vi "JoystickReader.vi"(8 "Reset":bool, 11 "Refnum in":refnum<k20>) -> (0 "L4 [deg]":sgl, 1 "L3 [0~100]":sgl, 2 "L2 [deg]":sgl, 3 "L1 [deg]":sgl)   [LabVIEW 2016]
uses:
  <vilib>/rvi/errors/niLvFpgaAdjustHostInterfaceError.vi
  <vilib>/Utility/error.llb/Error Cluster From Error Code.vi
  <vilib>/rvi/interface/nirviReadWriteControl/nirviReadWriteControl.xnode
  FPGA Bitfiles/IRISSControl_FPGATarget_IRISSFPGAIOv3.1_CU9txIsOgfM.lvbitx
  IRISS_FPGA_IO_v3.1.vi
  NiFpgaLv.dll
panel:
  in  "Joystick L4 home":i32
  in  "Joystick L3 home":i32
  in  "Joystick L2 home":i32
  in  "Joystick L1 home":i32
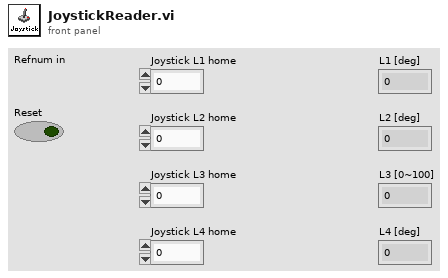
[diagram p1: front panel]
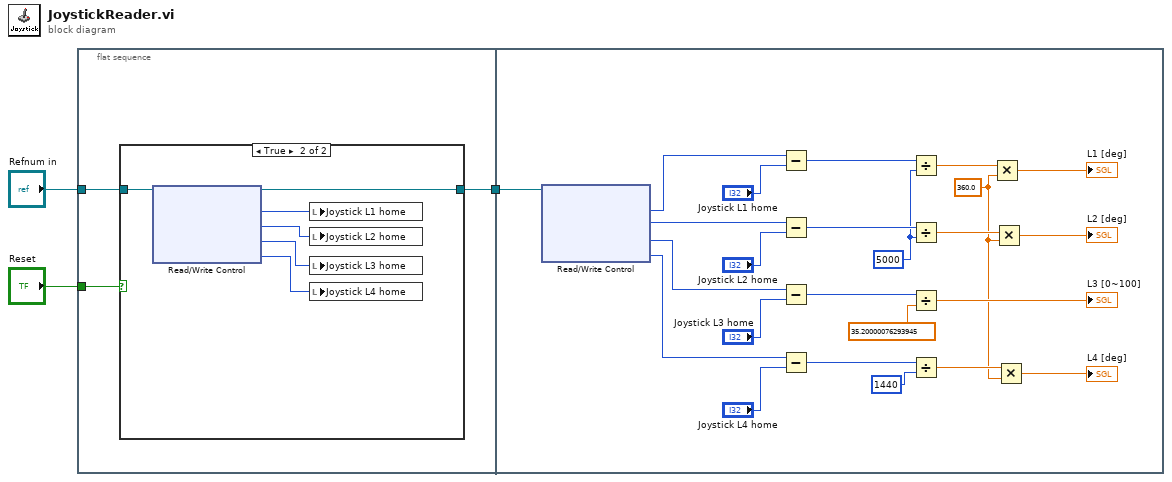
[diagram p0: block diagram]
diagram:
  n1 = flat-sequence {
    tunnel: "Refnum in" -> [w6]
    tunnel: [w5] -> w2
    tunnel: "Reset" -> [w4]
    tunnel: w2 -> [w14]
    frame #0 {
      n2 = case shown="True" w4 {
        tunnel: w6 -> [w7 w13]
        tunnel: [w7 w12] -> w5
        frame False {
        }
        frame True {
          n3 = xnode "Read/Write Control"("FPGA VI Reference In"=w13) -> ("FPGA VI Reference Out"=w12:refnum<k20>, "32 bit Position 9"=w11:i32, "32 bit Position 10"=w10:i32, "32 bit Position 11"=w9:i32, "32 bit Position 12"=w8:i32)  [unwired: 1 in, 1 out]
          n4 = local write "Joystick L1 home"(w11) -> ()
          n5 = local write "Joystick L2 home"(w10) -> ()
          n6 = local write "Joystick L3 home"(w9) -> ()
          n7 = local write "Joystick L4 home"(w8) -> ()
        }
      }
    }
    frame #1 {
      w18 = 360.0 ("y")
      w22 = 5000 ("y")
      n8 = xnode "Read/Write Control"("FPGA VI Reference In"=w14) -> ("32 bit Position 9"=w33:i32, "32 bit Position 10"=w32:i32, "32 bit Position 11"=w31:i32, "32 bit Position 12"=w30:i32)  [unwired: 1 in, 2 out]
      n9 = Subtract(x=w33, y="Joystick L1 home") -> (x-y=w29:i32)
      n10 = Subtract(x=w32, y="Joystick L2 home") -> (x-y=w28:i32)
      n11 = Subtract(x=w31, y="Joystick L3 home") -> (x-y=w27:i32)
      n12 = Subtract(x=w30, y="Joystick L4 home") -> (x-y=w26:i32)
      n13 = Divide(x=w29, y=w22) -> (x/y=w19:dbl)
      n14 = Divide(x=w28, y=w22) -> (x/y=w20:dbl)
      n15 = Divide(x=w27, y=sgl 35.2) -> (x/y=→"L3 [0~100]":sgl)
      n16 = Divide(x=w26, y=1440) -> (x/y=w21:dbl)
      n17 = Multiply(x=w19, y=w18) -> (x*y=→"L1 [deg]":dbl)
      n18 = Multiply(x=w20, y=w18) -> (x*y=→"L2 [deg]":dbl)
      n19 = Multiply(x=w21, y=w18) -> (x*y=→"L4 [deg]":dbl)
    }
  }
